vi "Send Remove View with Reply.vi"(7 "Priority":T1=enum."Normal" caption="Message Priority (Normal)", 8 "error in (no error)":errorcluster, 9 "timeout in ms (-1)":i32=-1, 10 "View":string, 11 "Message Enqueuer in":refnum<class "Message Enqueuer.lvclass">) -> (0 "error out":errorcluster, 3 "Message Enqueuer out":refnum<class "Message Enqueuer.lvclass">)   [LabVIEW 2017, in "GUI Views.lvlib" / "Remove View with Reply.lvclass"]
uses:
  Remove View with Reply.lvclass
  <vilib>/ActorFramework/Message Enqueuer/Message Priority.ctl
  <vilib>/ActorFramework/Message Enqueuer/Message Enqueuer.lvclass
  C:/Program Files/National Instruments/LabVIEW 2017/vi.lib/ActorFramework/Reply Msg/Reply Msg.lvclass
  Remove View with Reply.lvclass/Remove View with Reply.ctl
  <vilib>/ActorFramework/Reply Msg/Reply Msg.lvclass/Reply Msg.ctl
  <vilib>/ActorFramework/Message Enqueuer/Message Enqueuer.lvclass/Message Enqueuer.ctl
  <vilib>/ActorFramework/Message Enqueuer/Enqueue.vi
  <vilib>/ActorFramework/Reply Msg/Reply Msg.lvclass
  C:/Program Files/National Instruments/LabVIEW 2017/vi.lib/ActorFramework/Message/Message.lvclass
  <vilib>/Utility/LVClass/Get LV Class Name.vi
  <resource>/AFDebug/Generate Trace for Message.vi
  <vilib>/ActorFramework/Message Priority Queue/Priority Enqueue.vi
panel:
  out "Success":bool
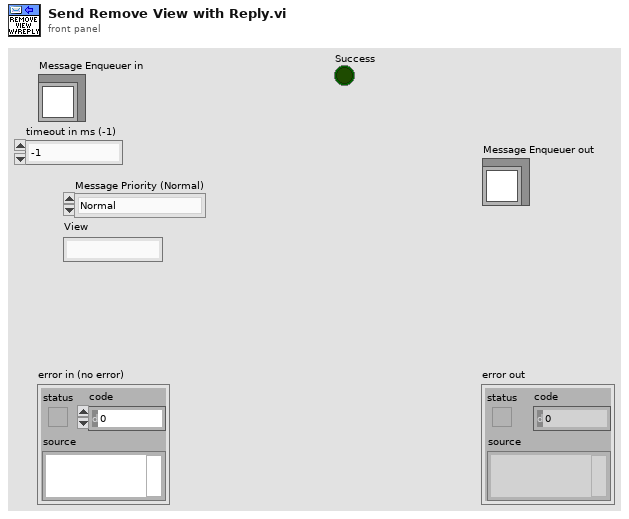
[diagram p1: front panel]
types:
  T1 = typedef "Actor Framework.lvlib/Message Enqueuer.lvclass/Message Priority.ctl" = enum16{"Low", "Normal", "High"}
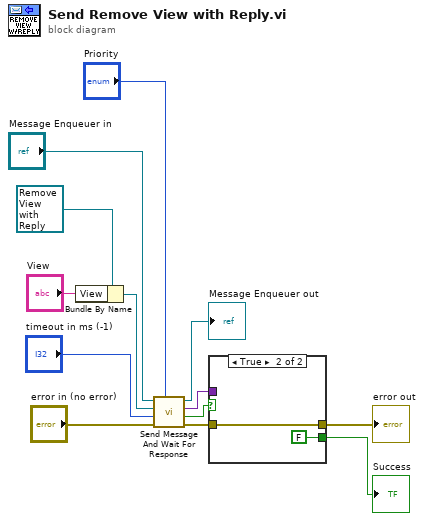
[diagram p0: block diagram]
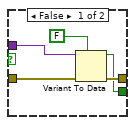
[diagram p2: hidden frame]
diagram:
  n1 = Bundle By Name(cluster=refnum<class "Remove View with Reply.lvclass"> refnum ("Remove View with Reply in"), "View"="View") -> (w6:refnum<class "Remove View with Reply.lvclass">)
  n2 = call <vilib>:"Send Message And Wait For Response.vi"("Message Priority (Normal)"="Priority", "error in (no error)"="error in (no error)", "timeout in ms (-1)"="timeout in ms (-1)", "Original Message"=w6, "Message Enqueuer in"="Message Enqueuer in") -> ("error out"=w5:errorcluster, "timed out?"=w2:bool, "Reply"=w3:variant, "Message Enqueuer out"=→"Message Enqueuer out":refnum<class "Message Enqueuer.lvclass">)  [unwired: 3 in]
  n3 = case shown="True" w2 {
    tunnel: w5 -> [w18 w20]
    tunnel: [w17 w20] -> w4
    tunnel: w3 -> [w15 _]
    tunnel: [w14 FALSE] -> w1
    frame False {
      n4 = Variant To Data(error in=w18, type=FALSE, Variant=w15) -> (data=w14:bool, error out=w17:errorcluster)
    }
    frame True {
    }
  }
  "error out" <- w4
  "Success" <- w1
